vi "OnSelect.vi"(8 "error in (no error)":errorcluster, 11 "MainMenu in":refnum<class "MainMenu.lvclass">) -> (0 "error out":errorcluster, 3 "MainMenu out":refnum<class "MainMenu.lvclass">)   [LabVIEW 2019, in "RT_Game.lvlib" / "MainMenu.lvclass"]
uses:
  MainMenu.lvclass
  C:/Users/FreshBob/Dropbox/VIs/myRIO_GameConsole/RT/RT_Game/Menu/Menu.lvclass
  C:/Users/FreshBob/Dropbox/VIs/myRIO_GameConsole/RT/RT_Game/Game/Game.lvclass
  Menu/Menu.lvclass/Menu.ctl
  MainMenu.lvclass/MainMenu.ctl
  Game/Game.lvclass/Game.ctl
  Menu/Read Selection.vi
  Game/Write SwitchGame.vi
  Game/Write FlattenedNextClass.vi
  Menu/Menu.lvclass
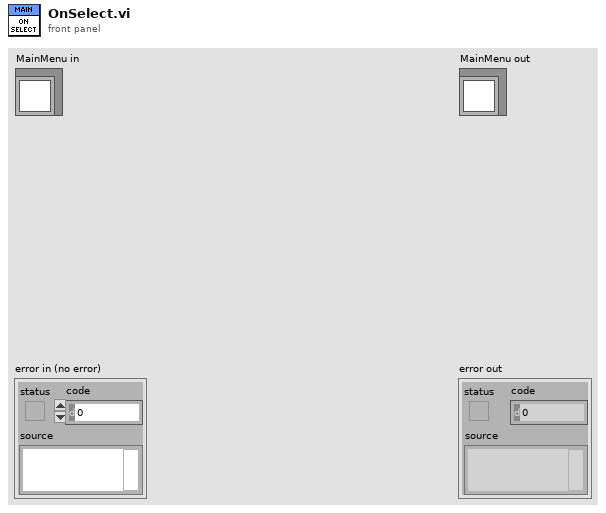
[diagram p1: front panel]
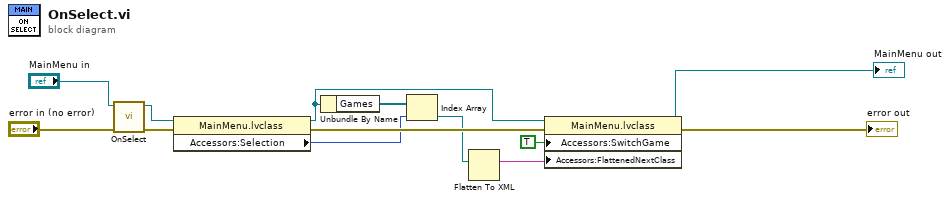
[diagram p0: block diagram]
diagram:
  n1 = call-parent "OnSelect.vi"("error in (no error)"="error in (no error)", "Menu in"="MainMenu in") -> ("error out"=w13:errorcluster, "Menu out"=w9:refnum<class "MainMenu.lvclass">)  [unwired: 8 in]
  n2 = property class="MainMenu.lvclass"(reference=w9, error in=w13) -> (reference out=w4:refnum<class "MainMenu.lvclass">, error out=w10:errorcluster, "Accessors:Selection"=w7:i8)
  n3 = Unbundle By Name(w4) -> ("Games"=w8:refnum<class "Game.lvclass">[])
  n4 = Index Array(array=w8, index=w7) -> (element=w2:refnum<class "Game.lvclass">)
  n5 = Flatten To XML(anything=w2) -> (xml string=w1:string)
  n6 = property class="MainMenu.lvclass"(reference=w4, error in=w10, "Accessors:SwitchGame"=TRUE ("SwitchGame_"), "Accessors:FlattenedNextClass"=w1) -> (reference out=→"MainMenu out":refnum<class "MainMenu.lvclass">, error out=→"error out":errorcluster)
